vi "Draw Robot.vi"(7 "Gyro":dbl, 10 "XY":cluster{"X":dbl, "Y":dbl}) -> (2 "Graph 2":cluster{cluster{"X":dbl, "Y":dbl}[]}[](graph))   [LabVIEW 2018]
panel:
  in  "Robot Lenght":dbl=32.0
  in  "Robot Width":dbl=28.0
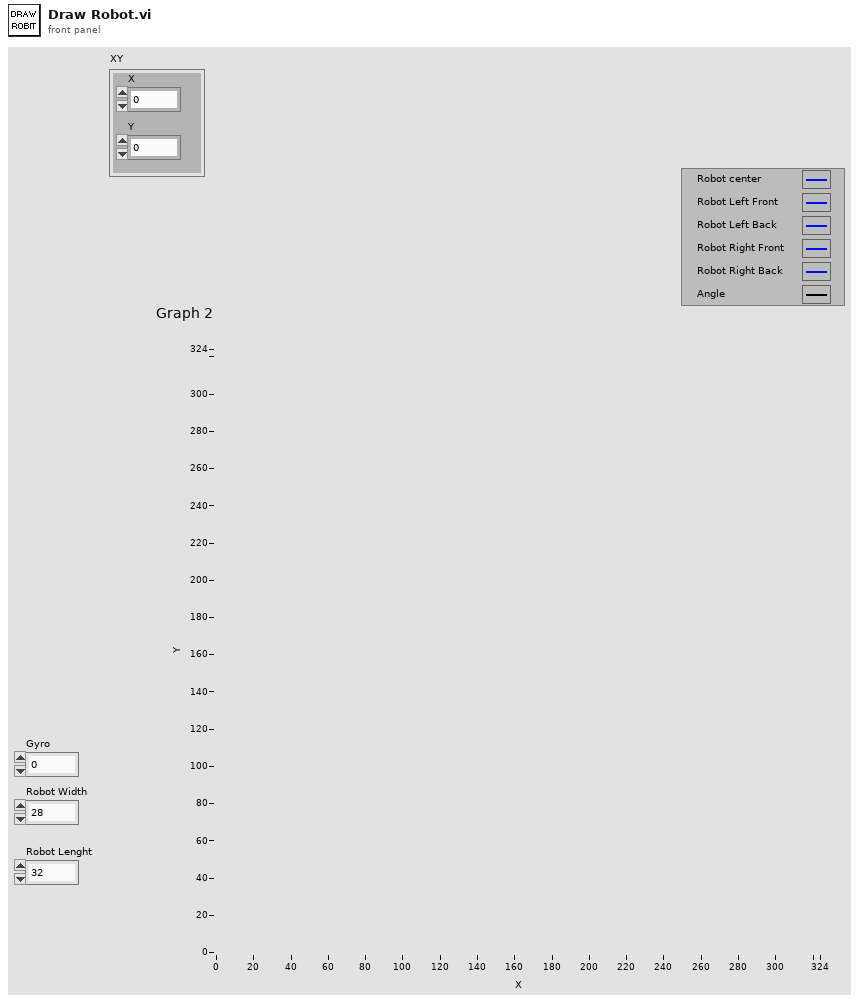
[diagram p1: front panel]
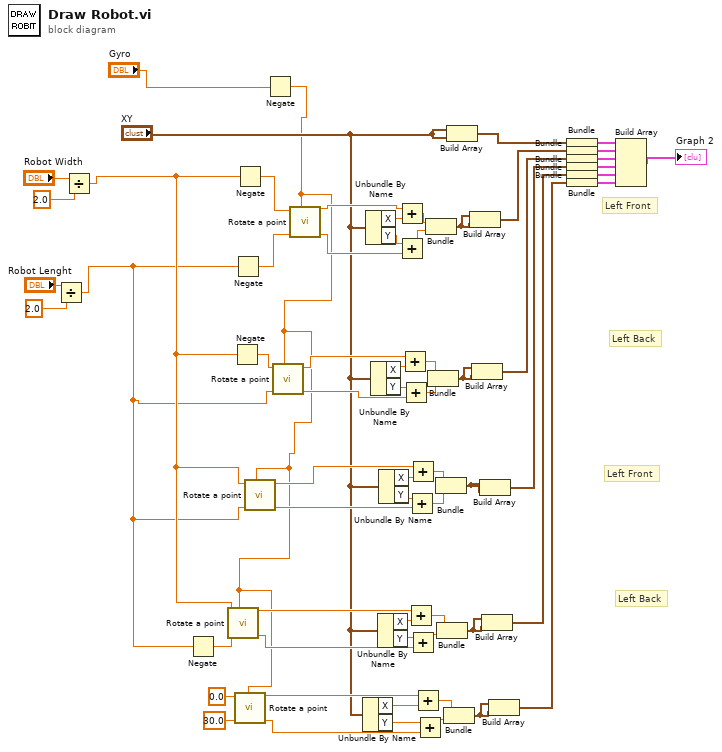
[diagram p0: block diagram]
diagram:
  # "Left Back"
  # "Left Front"
  # "Left Back"
  # "Left Front"
  n1 = Divide(x="Robot Lenght", y=2.0) -> (x/y=w43:dbl)
  n2 = Divide(x="Robot Width", y=2.0) -> (x/y=w44:dbl)
  n3 = Negate(x=w43) -> (-x=w48:dbl)
  n4 = Negate(x=w44) -> (-x=w45:dbl)
  n5 = Negate(x=w43) -> (-x=w46:dbl)
  n6 = Negate(x=w44) -> (-x=w47:dbl)
  n7 = Negate(x="Gyro") -> (-x=w2:dbl)
  n8 = call "Rotate a point.vi"("Gyro"=w2, "Y"=w48, "X"=w44) -> ("Y'"=w19:dbl, "X'"=w20:dbl)  [unwired: 7 in]
  n9 = call "Rotate a point.vi"("Gyro"=w2, "Y"=30.0, "X"=0.0) -> ("Y'"=w14:dbl, "X'"=w13:dbl)  [unwired: 7 in]
  n10 = call "Rotate a point.vi"("Gyro"=w2, "Y"=w43, "X"=w44) -> ("Y'"=w21:dbl, "X'"=w22:dbl)  [unwired: 7 in]
  n11 = call "Rotate a point.vi"("Gyro"=w2, "Y"=w43, "X"=w45) -> ("Y'"=w31:dbl, "X'"=w32:dbl)  [unwired: 7 in]
  n12 = call "Rotate a point.vi"("Gyro"=w2, "Y"=w46, "X"=w47) -> ("Y'"=w37:dbl, "X'"=w38:dbl)  [unwired: 7 in]
  n13 = Unbundle By Name("XY") -> ("X"=w7:dbl, "Y"=w6:dbl)
  n14 = Unbundle By Name("XY") -> ("X"=w42:dbl, "Y"=w41:dbl)
  n15 = Unbundle By Name("XY") -> ("X"=w35:dbl, "Y"=w34:dbl)
  n16 = Unbundle By Name("XY") -> ("X"=w25:dbl, "Y"=w23:dbl)
  n17 = Unbundle By Name("XY") -> ("X"=w30:dbl, "Y"=w27:dbl)
  n18 = Add(x=w38, y=w42) -> (x+y=w39:dbl)
  n19 = Add(x=w41, y=w37) -> (x+y=w40:dbl)
  n20 = Add(x=w32, y=w35) -> (x+y=w36:dbl)
  n21 = Add(x=w34, y=w31) -> (x+y=w33:dbl)
  n22 = Add(x=w20, y=w25) -> (x+y=w26:dbl)
  n23 = Add(x=w27, y=w21) -> (x+y=w29:dbl)
  n24 = Add(x=w22, y=w30) -> (x+y=w28:dbl)
  n25 = Add(x=w23, y=w19) -> (x+y=w24:dbl)
  n26 = Add(x=w13, y=w7) -> (x+y=w11:dbl)
  n27 = Add(x=w6, y=w14) -> (x+y=w12:dbl)
  n28 = Bundle(w39, w40) -> (w60:cluster{dbl, dbl})  [unwired: 1 in]
  n29 = Bundle(w36, w33) -> (w59:cluster{dbl, dbl})  [unwired: 1 in]
  n30 = Bundle(w28, w29) -> (w56:cluster{dbl, dbl})  [unwired: 1 in]
  n31 = Bundle(w26, w24) -> (w57:cluster{dbl, dbl})  [unwired: 1 in]
  n32 = Bundle(w11, w12) -> (w10:cluster{dbl, dbl})  [unwired: 1 in]
  n33 = Build Array("XY", "XY") -> (w62:cluster{"X":dbl, "Y":dbl}[])
  n34 = Build Array(w60, w60) -> (w61:cluster{dbl, dbl}[])
  n35 = Build Array(w59, w59) -> (w58:cluster{dbl, dbl}[])
  n36 = Build Array(w56, w56) -> (w55:cluster{dbl, dbl}[])
  n37 = Build Array(w57, w57) -> (w54:cluster{dbl, dbl}[])
  n38 = Build Array(w10, w10) -> (w8:cluster{dbl, dbl}[])
  n39 = Bundle(w62) -> (w63:cluster{cluster{"X":dbl, "Y":dbl}[]})  [unwired: 1 in]
  n40 = Bundle(w61) -> (w18:cluster{cluster{dbl, dbl}[]})  [unwired: 1 in]
  n41 = Bundle(w58) -> (w17:cluster{cluster{dbl, dbl}[]})  [unwired: 1 in]
  n42 = Bundle(w55) -> (w16:cluster{cluster{dbl, dbl}[]})  [unwired: 1 in]
  n43 = Bundle(w54) -> (w15:cluster{cluster{dbl, dbl}[]})  [unwired: 1 in]
  n44 = Bundle(w8) -> (w9:cluster{cluster{dbl, dbl}[]})  [unwired: 1 in]
  n45 = Build Array(w63, w18, w17, w16, w15, w9) -> (→"Graph 2":cluster{cluster{"X":dbl, "Y":dbl}[]}[])
